vi "Remove_LDA_Spikes.vi"(3 "Current Block Number":i32, 4 "Analaysis info Cluster":T1={"Colour"=0, "Inst type"=enum."Pitot-static tube", "Inst name"="Manometer voltage", "Symbol"="U", "Code name"="", "Extra Info"="U", "Inst Array"=enum."PWA", "Extra Titles"=[], "Extra Values"=[], "U"=0.0, "u^2"=0.0, "u^3"=0.0, "u^4"=0.0, "Skew_u"=0.0, "Kurt_u"=0.0, "Sd Error in Mean"=0.0, "% u'/U"=0.0, "X"=0.0, "Y"=0.0, "Z"=0.0, "Timescale integral Estimate"=0.0, "Sd Error in Variance"=0.0, "Calib File"=path "", "Calib Constants"=[], "Output Position"=FALSE, "Full Stats"=FALSE, "Av Sampling Rate"=0.0, "Av No of Samples"=0.0, "Total Meas Time (s)"=0.0, "ADAM Ch Name"="", "Max value"=0.0, "Min value"=0.0} {"Sd Error in Variance" format="%.2f"; "Skew_u" format="%.2f"; "% u'/U" format="%.2f"; "Sd Error in Mean" format="%.2f"; "Kurt_u" format="%.2f"; "u^4" format="%.2f"; "u^3" format="%.2f"; "U" format="%.2f"; "u^2" format="%.2f"}, 5 "Time Trace In":T4) -> (1 "Analaysis info Cluster Out":T1={"Colour"=0, "Inst type"=enum."Pitot-static tube", "Inst name"="Manometer voltage", "Symbol"="U", "Code name"="", "Extra Info"="U", "Inst Array"=enum."PWA", "Extra Titles"=[], "Extra Values"=[], "U"=0.0, "u^2"=0.0, "u^3"=0.0, "u^4"=0.0, "Skew_u"=0.0, "Kurt_u"=0.0, "Sd Error in Mean"=0.0, "% u'/U"=0.0, "X"=0.0, "Y"=0.0, "Z"=0.0, "Timescale integral Estimate"=0.0, "Sd Error in Variance"=0.0, "Calib File"=path "", "Calib Constants"=[], "Output Position"=FALSE, "Full Stats"=FALSE, "Av Sampling Rate"=0.0, "Av No of Samples"=0.0, "Total Meas Time (s)"=0.0, "ADAM Ch Name"="", "Max value"=0.0, "Min value"=0.0} {"Sd Error in Variance" format="%.2f"; "Skew_u" format="%.2f"; "% u'/U" format="%.2f"; "Sd Error in Mean" format="%.2f"; "Kurt_u" format="%.2f"; "u^4" format="%.2f"; "u^3" format="%.2f"; "U" format="%.2f"; "u^2" format="%.2f"}, 2 "Time trace Out":T4)   [LabVIEW 2016]
uses:
  Controls/Time_Trace_Cluster.ctl
  Controls/Analysis_info_cluster.ctl
  Controls/Inst_type.ctl
  Controls/Instrument_Array.ctl
  Globals/Meas_global.vi
  <vilib>/Analysis/NI_AALBase.lvlib
panel:
  out "After":cluster{"Time (s)":dbl[], "Eng Values":dbl[]}(graph)
  out "Before":cluster{"Time (s)":dbl[], "Eng Values":dbl[]}(graph)
  in  "Display plots":bool
  out "x-y":i32
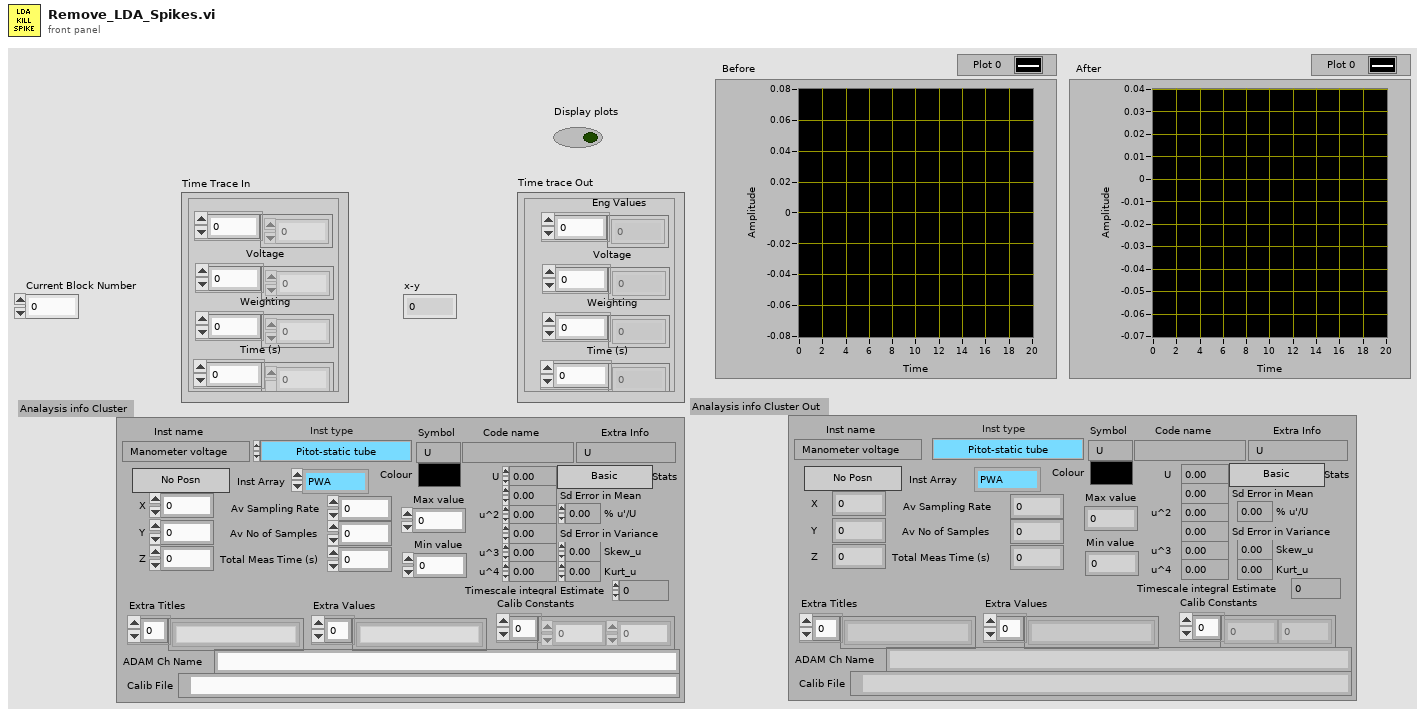
[diagram p1: front panel]
types:
  T1 = typedef "Analysis_info_cluster.ctl" = cluster{"Colour":u32, "Inst type":T2, "Inst name":string, "Symbol":string, "Code name":string, "Extra Info":string, "Inst Array":T3, "Extra Titles":string[], "Extra Values":string[], "U":dbl, "u^2":dbl, "u^3":dbl, "u^4":dbl, "Skew_u":dbl, "Kurt_u":dbl, "Sd Error in Mean":dbl, "% u'/U":dbl, "X":dbl, "Y":dbl, "Z":dbl, "Timescale integral Estimate":dbl, "Sd Error in Variance":dbl, "Calib File":path, "Calib Constants":dbl[], "Output Position":bool, "Full Stats":bool, "Av Sampling Rate":dbl, "Av No of Samples":dbl, "Total Meas Time (s)":dbl, "ADAM Ch Name":string, "Max value":dbl, "Min value":dbl}
  T2 = typedef "Inst_type.ctl" = enum16{"Propeller anemometer", "Raw voltage", "Pressure Transducer", "Pitot-static tube", "Preston tube", "Hot wire", "Cross wire 1", "Cross wire 2", "Generic Linear", "Generic Polynomial", "Generic BackPoly", "Fast FID", "Thermocouple", "Cold wire", "Pulsed Wire", "LDA Vel", "LDA Tran time", "LDA Arr time", "Microphone"}
  T3 = typedef "Instrument_Array.ctl" = enum16{"PWA", "LDA", "Analogue"}
  T4 = typedef "Time_Trace_Cluster.ctl" = cluster{"Weighting":dbl[], "Time (s)":dbl[], "Voltage":dbl[], "Eng Values":dbl[]}
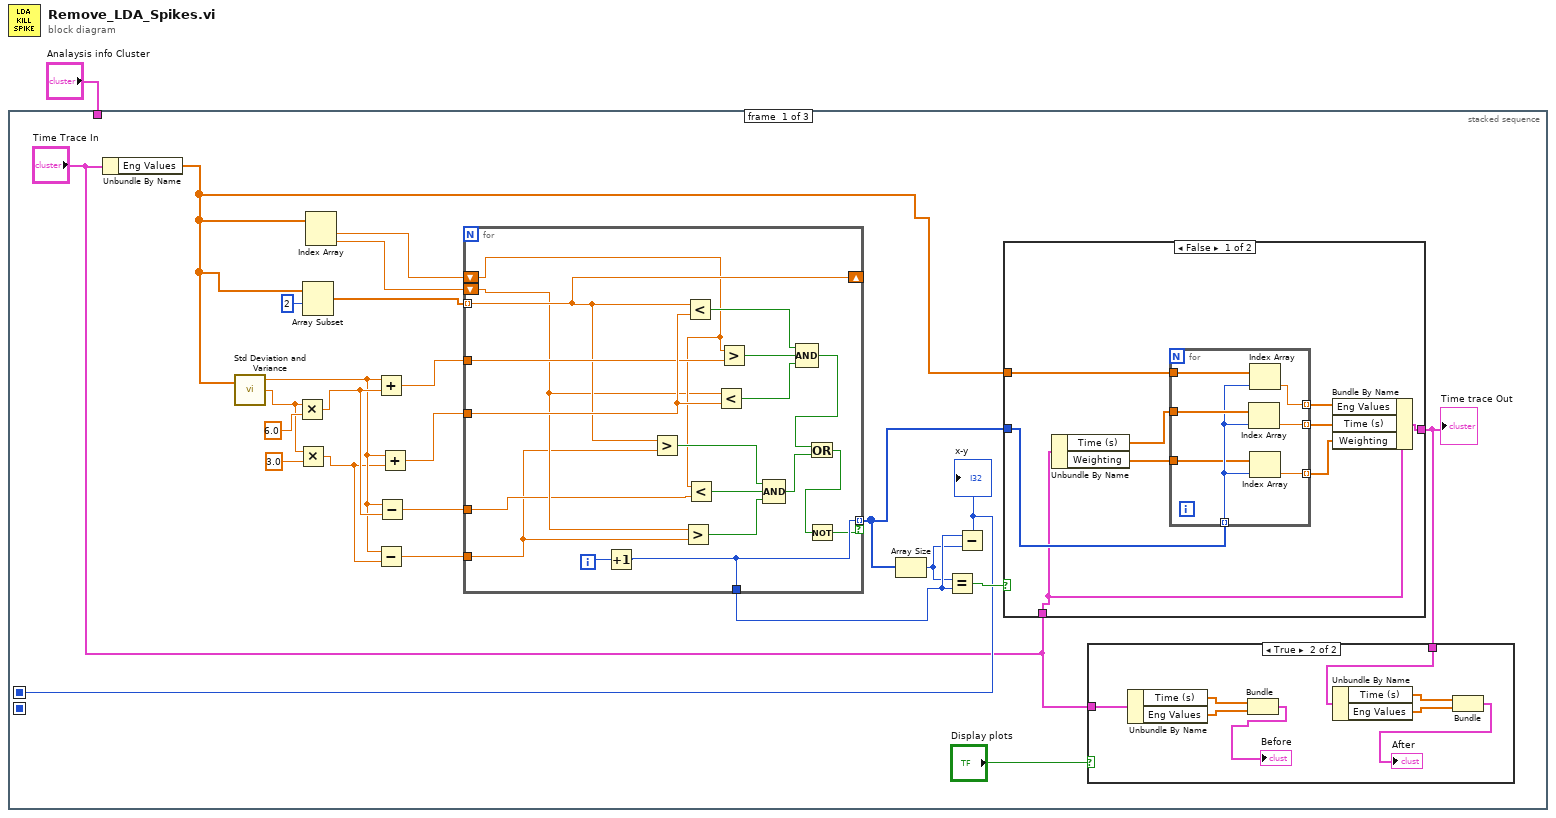
[diagram p0: block diagram]
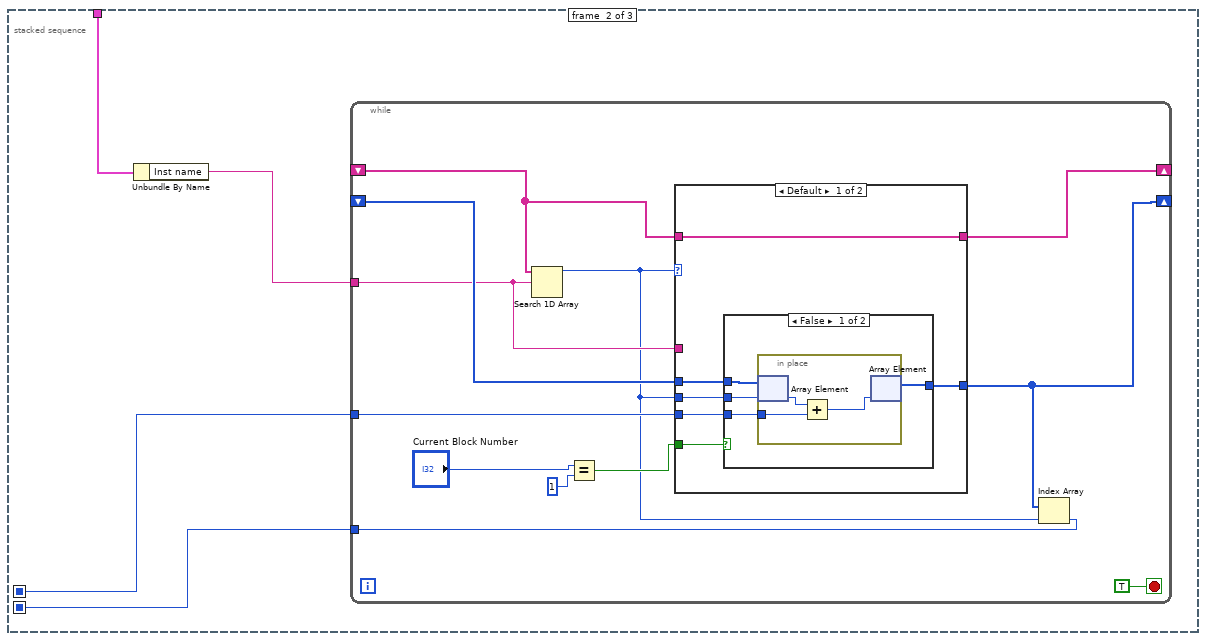
[diagram p4: hidden frame]
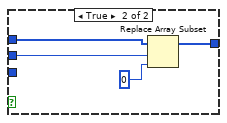
[diagram p5: hidden frame]
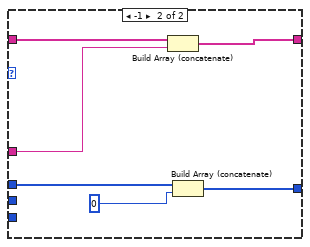
[diagram p6: hidden frame]
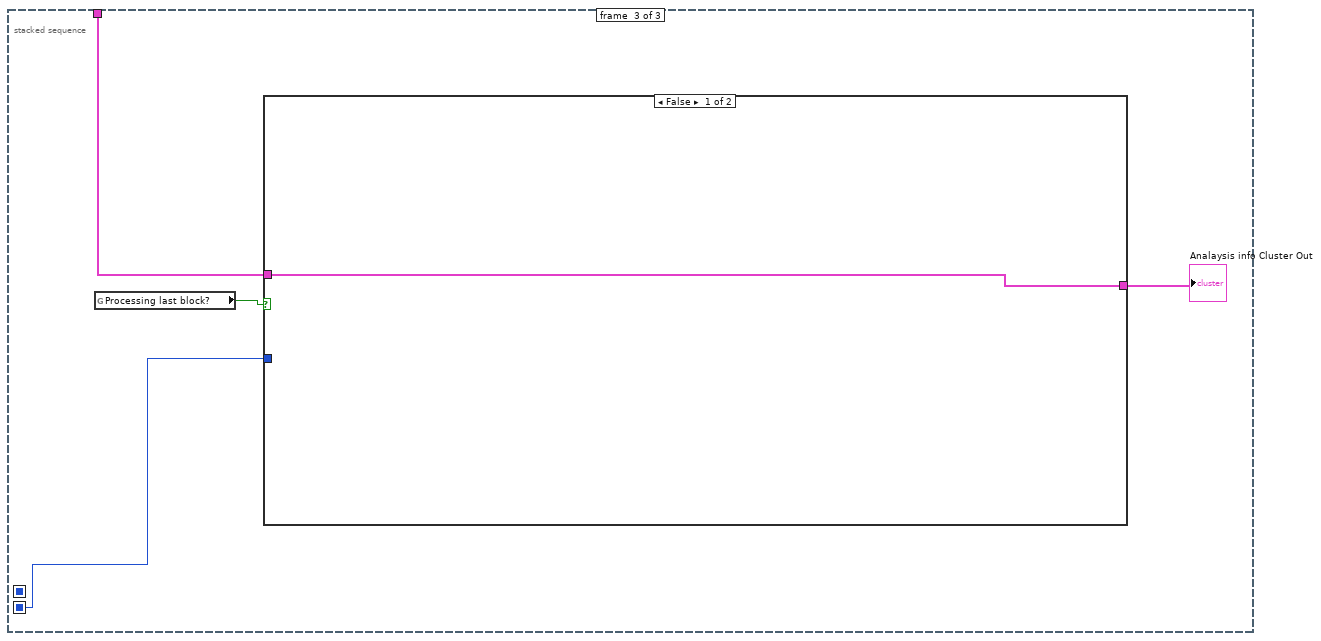
[diagram p7: hidden frame]
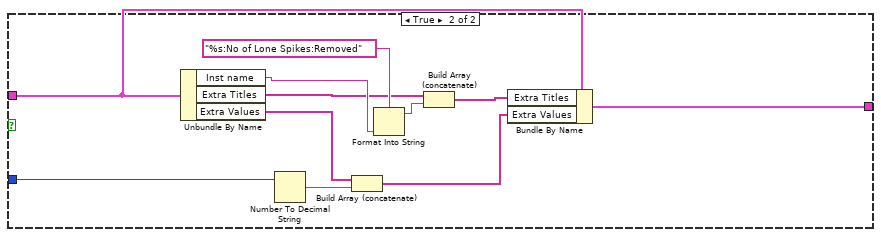
[diagram p8: hidden frame]
diagram:
  n1 = stacked-sequence {
    seq-local: [w10 _ _] -> [_ w72 _]
    seq-local: [_ w69 _] -> [_ _ w108]
    tunnel: "Analaysis info Cluster" -> [_ w71 w110]
    frame #0 {
      n2 = Unbundle By Name("Time Trace In") -> ("Eng Values"=w13:dbl[])
      n3 = call <vilib>:"Std Deviation and Variance.vi"("X"=w13) -> ("mean"=w8:dbl, "standard deviation"=w21:dbl)  [unwired: 1 in, 1 out]
      n4 = Multiply(x=w21, y=6.0) -> (x*y=w9:dbl)
      n5 = Multiply(x=w21, y=3.0) -> (x*y=w7:dbl)
      n6 = Array Subset(array=w13, index=2) -> (w16:dbl[])  [unwired: 1 in]
      n7 = Index Array(array=w13) -> (element #1=w19:dbl, element #2=w18:dbl)  [unwired: 2 in]
      n8 = Add(x=w8, y=w9) -> (x+y=w23:dbl)
      n9 = Subtract(x=w8, y=w7) -> (x-y=w5:dbl)
      n10 = Subtract(x=w8, y=w9) -> (x-y=w6:dbl)
      n11 = Add(x=w8, y=w7) -> (x+y=w20:dbl)
      n12 = for {
        tunnel: w23 -> [w67]
        tunnel: w16 -> [w58] mode=indexing
        shift-right: [w58] -> _
        shift-left: w19 -> [w57]
        shift-left: w18 -> [w56]
        tunnel: w20 -> [w68]
        tunnel: [w62] -> w14 mode=indexing if=w51
        tunnel: [w62] -> w12
        tunnel: w6 -> [w55]
        tunnel: w5 -> [w54]
        i -> [w63]
        n13 = Increment(x=w63) -> (x+1=w62:i32)
        n14 = Greater?(x=w58, y=w54) -> (0:w59:bool)
        n15 = Greater?(x=w56, y=w54) -> (0:w61:bool)
        n16 = Less?(x=w58, y=w68) -> (x < y?=w66:bool)
        n17 = Less?(x=w57, y=w55) -> (x < y?=w60:bool)
        n18 = Less?(x=w56, y=w68) -> (x < y?=w64:bool)
        n19 = Greater?(x=w57, y=w67) -> (0:w65:bool)
        n20 = Compound Arithmetic op=AND(w59, w60, w61) -> (w53:bool)
        n21 = Compound Arithmetic op=AND(w66, w65, w64) -> (w52:bool)
        n22 = Or(x=w52, y=w53) -> (x .or. y?=w50:bool)
        n23 = Not(x=w50) -> (.not. x?=w51:bool)
      }
      n24 = Array Size(array=w14) -> (size(s)=w11:i32)
      n25 = Equal?(x=w11, y=w12) -> (x = y?=w15:bool)
      n26 = Subtract(x=w12, y=w11) -> (x-y=w10:i32)
      "x-y" <- w10
      n27 = case shown="False" w15 {
        tunnel: [w36 w49] -> w2
        tunnel: "Time Trace In" -> [w37 w49]
        tunnel: w14 -> [w41 _]
        tunnel: w13 -> [w38 _]
        frame False {
          n28 = Unbundle By Name(w37) -> ("Time (s)"=w40:dbl[], "Weighting"=w39:dbl[])
          n29 = for {
            tunnel: w41 -> [w44] mode=indexing
            tunnel: w38 -> [w48]
            tunnel: w40 -> [w47]
            tunnel: [w46] -> w35 mode=indexing
            tunnel: [w45] -> w34 mode=indexing
            tunnel: w39 -> [w43]
            tunnel: [w42] -> w33 mode=indexing
            n30 = Index Array(array=w47, index=w44) -> (element=w45:dbl)
            n31 = Index Array(array=w48, index=w44) -> (element=w46:dbl)
            n32 = Index Array(array=w43, index=w44) -> (element=w42:dbl)
          }
          n33 = Bundle By Name(cluster=w37, "Eng Values"=w35, "Time (s)"=w34, "Weighting"=w33) -> (w36:T4)
        }
        frame True {
        }
      }
      "Time trace Out" <- w2
      n34 = case shown="True" "Display plots" {
        tunnel: "Time Trace In" -> [_ w32]
        tunnel: w2 -> [_ w27]
        frame False {
        }
        frame True {
          n35 = Unbundle By Name(w32) -> ("Time (s)"=w31:dbl[], "Eng Values"=w30:dbl[])
          n36 = Bundle("Time (s)"=w31, "Eng Values"=w30) -> (→"Before":cluster{"Time (s)":dbl[], "Eng Values":dbl[]})  [unwired: 1 in]
          n37 = Unbundle By Name(w27) -> ("Time (s)"=w28:dbl[], "Eng Values"=w29:dbl[])
          n38 = Bundle("Time (s)"=w28, "Eng Values"=w29) -> (→"After":cluster{"Time (s)":dbl[], "Eng Values":dbl[]})  [unwired: 1 in]
        }
      }
    }
    frame #1 {
      n39 = Unbundle By Name(w71) -> ("Inst name"=w70:string)
      n40 = while {
        tunnel: w70 -> [w80]
        shift-right: [w83] -> _
        shift-left: _ -> [w81]
        shift-right: [w75] -> _
        shift-left: _ -> [w82]
        tunnel: w72 -> [w78]
        tunnel: [w73] -> w69
        stop <- TRUE stop-if-true
        n41 = Search 1D Array(1D array=w81, element=w80) -> (index of element=w74:i32)  [unwired: 1 out]
        n42 = Equal?(x="Current Block Number", y=1) -> (x = y?=w76:bool)
        n43 = case shown="Default" w74 {
          tunnel: w81 -> [w90 w107]
          tunnel: w80 -> [_ w106]
          tunnel: [w90 w105] -> w83
          tunnel: w82 -> [w89 w104]
          tunnel: [w88 w103] -> w75
          tunnel: w74 -> [w87 _]
          tunnel: w76 -> [w86 _]
          tunnel: w78 -> [w85 _]
          frame Default {
            n44 = case shown="False" w86 {
              tunnel: w89 -> [w93 w101]
              tunnel: [w91 w100] -> w88
              tunnel: w87 -> [w94 w99]
              tunnel: w85 -> [w92 _]
              frame False {
                n45 = in-place {
                  in-place-border: w92 -> [w96]
                  n46 = in-place-array #1(w93, w94) -> (w97:i32)
                  n47 = Add(x=w97, y=w96) -> (x+y=w95:i32)
                  n48 = in-place-array #1(w95) -> (w91:i32[])  [unwired: 1 out]
                }
              }
              frame True {
                n49 = Replace Array Subset(array=w101, new element=0, index=w99) -> (w100:i32[])
              }
            }
          }
          frame -1 {
            n50 = Build Array (concatenate)(w107, w106) -> (w105:string[])
            n51 = Build Array (concatenate)(w104, 0) -> (w103:i32[])
          }
        }
        n52 = Index Array(array=w75, index=w74) -> (element=w73:i32)
      }
    }
    frame #2 {
      n53 = global read "Meas_global.vi" "Processing last block?"() -> (w111:bool)
      n54 = case shown="False" w111 {
        tunnel: w110 -> [w112 w114]
        tunnel: [w112 w115] -> w109
        tunnel: w108 -> [_ w113]
        frame False {
        }
        frame True {
          n55 = Unbundle By Name(w114) -> ("Inst name"=w122:string, "Extra Titles"=w118:string[], "Extra Values"=w119:string[])
          n56 = Number To Decimal String(number=w113) -> (decimal integer string=w116:string)  [unwired: 1 out]
          n57 = Build Array (concatenate)(w119, w116) -> (w120:string[])
          n58 = Format Into String(format string="%s:No of Lone Spikes:Removed", w122) -> (resulting string=w121:string)  [unwired: 2 in, 1 out]
          n59 = Build Array (concatenate)(w118, w121) -> (w117:string[])
          n60 = Bundle By Name(cluster=w114, "Extra Titles"=w117, "Extra Values"=w120) -> (w115:T1)
        }
      }
      "Analaysis info Cluster Out" <- w109
    }
  }
